vi "Remove_First_Point.vi"(8 "error in":errorcluster caption="entrée d'erreur", 11 "Data_AI":dbl[](array[numeric])=[1.0, 2.0, 3.0, 4.0, 5.0, 6.0, 7.0, 8.0]) -> (0 "error out":errorcluster caption="sortie d'erreur", 3 "Data_AI out":dbl[](array[numeric])=[1.0, 2.0, 3.0, 4.0, 5.0, 6.0, 7.0, 8.0])   [LabVIEW 2026]
panel:
  out "Size OUT":i32
  out "Size IN":i32
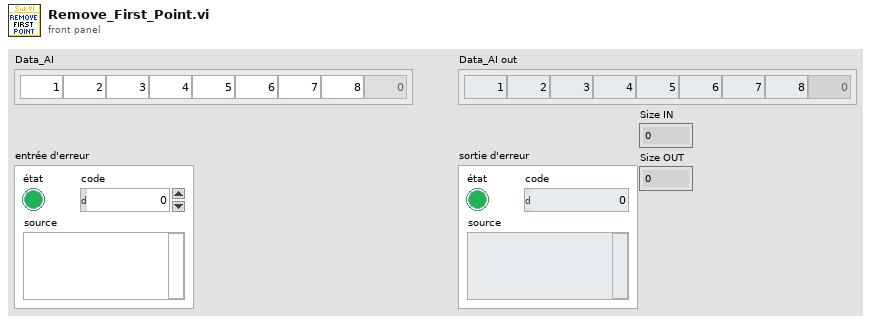
[diagram p1: front panel]
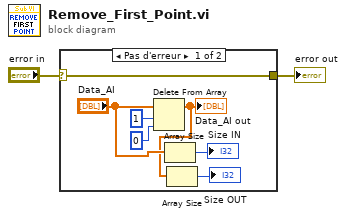
[diagram p0: block diagram]
diagram:
  n1 = case shown="Pas d'erreur" "error in" {
    selector: "error in" -> [w7 w10]
    tunnel: [w7 w10] -> w1
    frame No Error {
      n2 = Delete From Array(array="Data_AI", length=1 ("longueur"), index=0 ("indice")) -> (array with subset deleted=w4:dbl[])  [unwired: 1 out]
      "Data_AI out" <- w4
      n3 = Array Size(array="Data_AI") -> (size(s)=→"Size IN":i32)
      n4 = Array Size(array=w4) -> (size(s)=→"Size OUT":i32)
    }
    frame Error {
    }
  }
  "error out" <- w1
